vi "Dequeue Enum.vi"(8 "error in":errorcluster, 9 "Timeout State (0)":i32, 10 "Timeout ms (-1)":i32=-1, 11 "Queue In":refnum<queue>) -> (0 "error out":errorcluster, 1 "Data":variant, 2 "State":i32, 3 "Queue Out":refnum<queue>)   [LabVIEW 2020, in "Enum Queue State Machine.lvlib"]
uses:
  Enum Queue State Machine.lvlib
  Controls/Enum Message.ctl
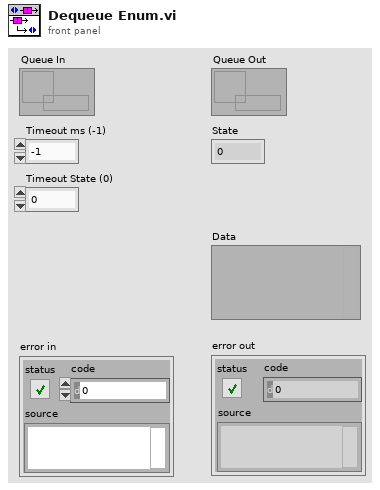
[diagram p1: front panel]
types:
  T1 = typedef "Enum Queue State Machine.lvlib/Enum Message.ctl" = cluster{"State":i32, "Data":variant}
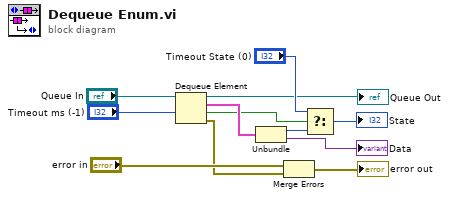
[diagram p0: block diagram]
diagram:
  n1 = Dequeue Element(queue="Queue In", timeout in ms (-1)="Timeout ms (-1)") -> (queue out=→"Queue Out":refnum<queue>, element=w11:T1, timed out?=w7:bool, error out=w8:errorcluster)  [unwired: 1 in]
  n2 = Unbundle(w11) -> ("State"=w6:i32, "Data"=→"Data":variant)
  n3 = Merge Errors("error in", w8) -> (→"error out":errorcluster)
  n4 = Select(t="Timeout State (0)", s=w7, f=w6) -> (s? t:f=→"State":i32)
